vi "subvi_readjpg.vi"(8 "Cluster":T1, 11 "length":i32) -> (0 "image size y":i32, 1 "image size x":i32, 2 "image subset y":i32, 3 "image subset x":i32, 5 "image data":T2)   [LabVIEW 2014]
uses:
  <vilib>/picture/picture.llb/imagedata.ctl
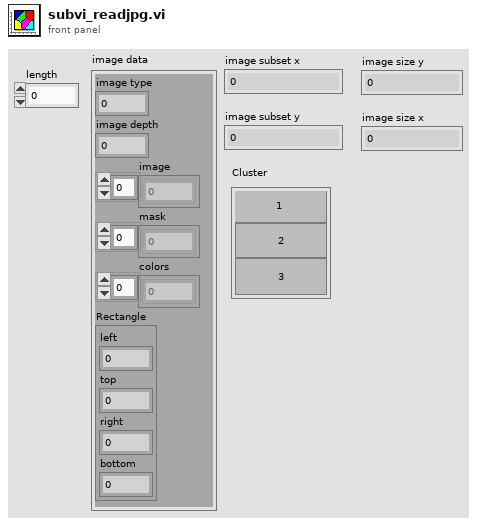
[diagram p1: front panel]
types:
  T1 = cluster{"OK Button":bool, "OK Button 2":bool, "OK Button 3":bool}
  T2 = typedef "imagedata.ctl" = cluster{"image type":i32, "image depth":i32, "image":u8[], "mask":u8[], "colors":u32[], "Rectangle":cluster{"left":i16, "top":i16, "right":i16, "bottom":i16}}
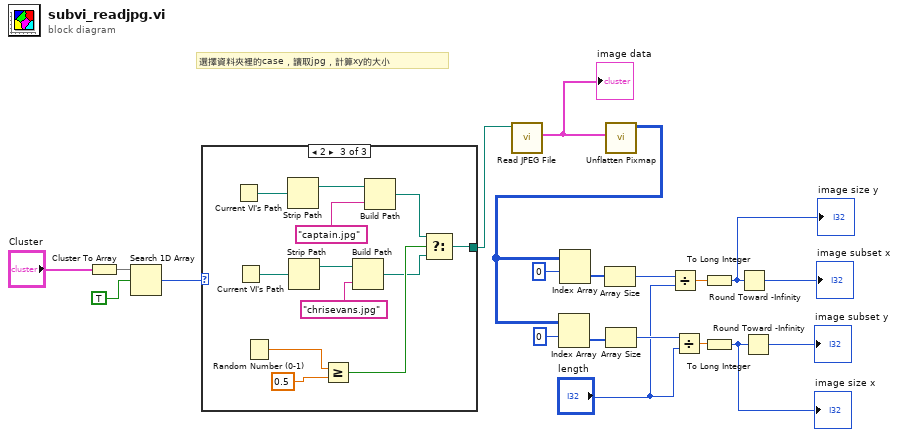
[diagram p0: block diagram]
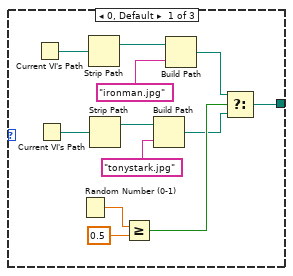
[diagram p2: hidden frame]
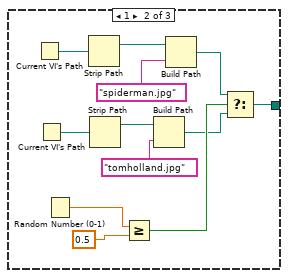
[diagram p3: hidden frame]
diagram:
  # "選擇資料夾裡的case，讀取jpg，計算xy的大小"
  n1 = Cluster To Array(cluster="Cluster") -> (array=w20:bool[])
  n2 = Search 1D Array(1D array=w20, element=TRUE) -> (index of element=w18:i32)  [unwired: 1 in]
  n3 = case shown="2" w18 {
    tunnel: [w21 w33 w45] -> w17
    frame 0, Default {
      n4 = Current VI's Path() -> (path=w29:path)
      n5 = Current VI's Path() -> (path=w25:path)
      n6 = Random Number (0-1)() -> (number: 0 to 1=w32:dbl)
      n7 = Strip Path(path=w29) -> (stripped path=w28:path)  [unwired: 1 out]
      n8 = Strip Path(path=w25) -> (stripped path=w24:path)  [unwired: 1 out]
      n9 = Greater Or Equal?(x=w32, y=0.5) -> (x >= y?=w30:bool)
      n10 = Build Path(base path=w24, name or relative path="tonystark.jpg") -> (appended path=w22:path)
      n11 = Build Path(base path=w28, name or relative path="ironman.jpg") -> (appended path=w26:path)
      n12 = Select(t=w26, s=w30, f=w22) -> (s? t:f=w21:path)
    }
    frame 1 {
      n13 = Current VI's Path() -> (path=w41:path)
      n14 = Current VI's Path() -> (path=w37:path)
      n15 = Random Number (0-1)() -> (number: 0 to 1=w44:dbl)
      n16 = Strip Path(path=w41) -> (stripped path=w40:path)  [unwired: 1 out]
      n17 = Strip Path(path=w37) -> (stripped path=w36:path)  [unwired: 1 out]
      n18 = Greater Or Equal?(x=w44, y=0.5) -> (x >= y?=w42:bool)
      n19 = Build Path(base path=w36, name or relative path="tomholland.jpg") -> (appended path=w34:path)
      n20 = Build Path(base path=w40, name or relative path="spiderman.jpg") -> (appended path=w38:path)
      n21 = Select(t=w38, s=w42, f=w34) -> (s? t:f=w33:path)
    }
    frame 2 {
      n22 = Current VI's Path() -> (path=w53:path)
      n23 = Current VI's Path() -> (path=w49:path)
      n24 = Random Number (0-1)() -> (number: 0 to 1=w56:dbl)
      n25 = Strip Path(path=w53) -> (stripped path=w52:path)  [unwired: 1 out]
      n26 = Strip Path(path=w49) -> (stripped path=w48:path)  [unwired: 1 out]
      n27 = Greater Or Equal?(x=w56, y=0.5) -> (x >= y?=w54:bool)
      n28 = Build Path(base path=w48, name or relative path="chrisevans.jpg") -> (appended path=w46:path)
      n29 = Build Path(base path=w52, name or relative path="captain.jpg") -> (appended path=w50:path)
      n30 = Select(t=w50, s=w54, f=w46) -> (s? t:f=w45:path)
    }
  }
  n31 = call <vilib>:"Read JPEG File.vi"("path to JPEG file"=w17) -> ("image data"=w16:T2)  [unwired: 8 in, 2 out]
  "image data" <- w16
  n32 = call <vilib>:"Unflatten Pixmap.vi"("image data"=w16) -> ("24-bit pixmap"=w3:u32[][])  [unwired: 4 in, 6 out]
  n33 = Index Array(array=w3, index (row)=0) -> (element=w12:u32[])  [unwired: 1 in]
  n34 = Index Array(array=w3, index (row)=0) -> (element=w13:u32[])  [unwired: 1 in]
  n35 = Array Size(array=w13) -> (size(s)=w11:i32)
  n36 = Array Size(array=w12) -> (size(s)=w10:i32)
  n37 = Divide(x=w11, y="length") -> (x/y=w8:dbl)
  n38 = Divide(x=w10, y="length") -> (x/y=w7:dbl)
  n39 = To Long Integer(number=w8) -> (32bit integer=w6:i32)
  "image size y" <- w6
  n40 = To Long Integer(number=w7) -> (32bit integer=w2:i32)
  "image size x" <- w2
  n41 = Round Toward -Infinity(1:w6) -> (0:→"image subset x":i32)
  n42 = Round Toward -Infinity(1:w2) -> (0:→"image subset y":i32)
